vi "16TVTI-Read.vi"(6 "Channel":i16, 7 "IO Info":T1={"Com Port"=1, "ISOBUS Address"=1, "GPIB Address"=1, "Communication"=enum."ISOBUS"}) -> (1 "Display Text":string="0", 2 "Temperature":dbl[unit] format="%.2f", 3 "ITC IO Info":T1={"Com Port"=1, "ISOBUS Address"=1, "GPIB Address"=1, "Communication"=enum."ISOBUS"})   [LabVIEW 2016]
doc: "Reads the actual temperature for the specified channel."
uses:
  Equipment/Oxford Software/Oxsoft/ITCSUBS.LLB/ITCIO.ctl
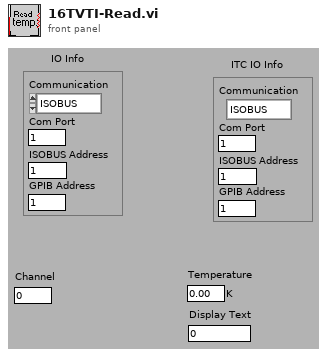
[diagram p1: front panel]
types:
  T1 = typedef "ITCIO.ctl" = cluster{"Com Port":i32, "ISOBUS Address":i32, "GPIB Address":i16, "Communication":enum16{"RS232", "ISOBUS", "GPIB", "Gateway"}}
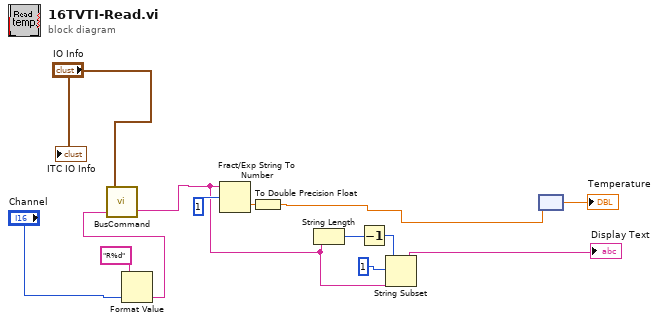
[diagram p0: block diagram]
diagram:
  n1 = Format Value(format string="R%d", value (0)="Channel") -> (output string=w8:string)  [unwired: 1 in]
  n2 = call "BusCommand.vi"("Command"=w8, "Instrument address (in)"="IO Info") -> ("Reply"=w7:string)  [unwired: 1 out]
  n3 = Fract/Exp String To Number(string=w7, offset=1) -> (number=w12:dbl)  [unwired: 2 in, 1 out]
  n4 = To Double Precision Float(number=w12) -> (double precision float=w11:dbl)
  n5 = String Length(string=w7) -> (length=w3:i32)
  n6 = Decrement(x=w3) -> (x-1=w2:i32)
  n7 = String Subset(string=w7, offset (0)=1, length (rest)=w2) -> (substring=→"Display Text":string)
  n8 = node(w11) -> (→"Temperature":dbl[unit])
  "ITC IO Info" <- "IO Info"
